vi "Free up serial number.vi"() -> ()   [LabVIEW 2013]
panel:
  in  "Serial number":string
  out "Error out":errorcluster
  in  "Error in (no error)":errorcluster
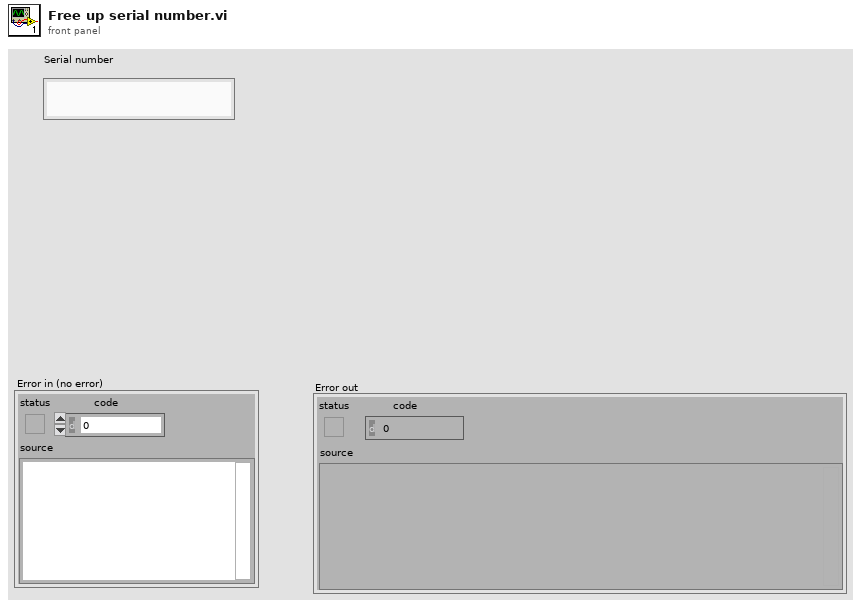
[diagram p1: front panel]
types:
  T1 = enum16{"Query", "Insert", "Select", "Dump Recs", "Get Rec Count", "Get Col Names", "Insert all fields", "Find", "Get last test result", "Get work order qty", "Set work order qty", "Save test report", "Get test report", "Execute query no data", "Select count", "Query and return row 0 col 0"}
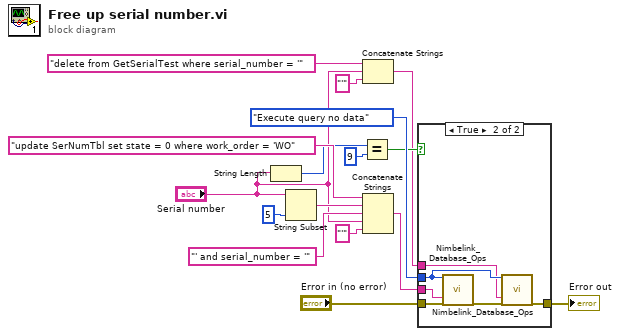
[diagram p0: block diagram]
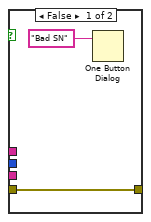
[diagram p2: hidden frame]
diagram:
  n1 = String Length(string="Serial number") -> (length=w7:i32)
  n2 = String Subset(string="Serial number", length (rest)=5 ("length (rest)")) -> (substring=w11:string)  [unwired: 1 in]
  n3 = Equal?(x=w7, y=9) -> (x = y?=w5:bool)
  n4 = Concatenate Strings("delete from GetSerialTest where serial_number = '" ("string"), "Serial number", "'" ("string")) -> (w1:string)
  n5 = Concatenate Strings("update SerNumTbl set state = 0 where work_order = 'WO" ("string"), w11, "' and serial_number = '" ("string"), "Serial number", "'" ("string")) -> (w8:string)
  n6 = case shown="True" w5 {
    tunnel: "Error in (no error)" -> [w18 w24]
    tunnel: [w18 w19] -> w15
    tunnel: T1."Execute query no data" ("Operation") -> [_ w21]
    tunnel: w8 -> [_ w23]
    tunnel: w1 -> [_ w20]
    frame False {
      n7 = One Button Dialog(message="Bad SN") -> ()  [unwired: 1 in, 1 out]
    }
    frame True {
      n8 = call "Nimbelink_Database_Ops.vi"("Operation"=w21, "SQL Query"=w23, "Error in (no error)"=w24) -> ("Error out"=w22:errorcluster)  [unwired: 9 in, 7 out]
      n9 = call "Nimbelink_Database_Ops.vi"("Operation"=w21, "SQL Query"=w20, "Error in (no error)"=w22) -> ("Error out"=w19:errorcluster)  [unwired: 9 in, 7 out]
    }
  }
  "Error out" <- w15
